vi "Get Installed Set Extended.vi"(8 "error in (no error)":errorcluster, 9 "Item Types (all visible)":T1 items=["all visible", "all including hidden", "standard only", "startup only"], 10 "Cached (F)":bool, 11 "Session in":refnum<k21>) -> (0 "error out":errorcluster, 2 "Software Set":T2 {"Items"."Visibility Type" items=["standard", "hidden", "system", "unknown", "startup", "image"]; "Add-ons"."Visibility Type" items=["standard", "hidden", "system", "unknown", "startup", "image"]}, 3 "Session out":refnum<k21>)   [LabVIEW 2012, in "nisyscfg.lvlib"]
uses:
  <vilib>/nisyscfg/nisyscfg.lvlib
  <vilib>/nisyscfg/Software Set Extended.ctl
  <vilib>/nisyscfg/Software Extended.ctl
  <vilib>/nisyscfg/Component Type.ctl
  <vilib>/nisyscfg/Component Types.ctl
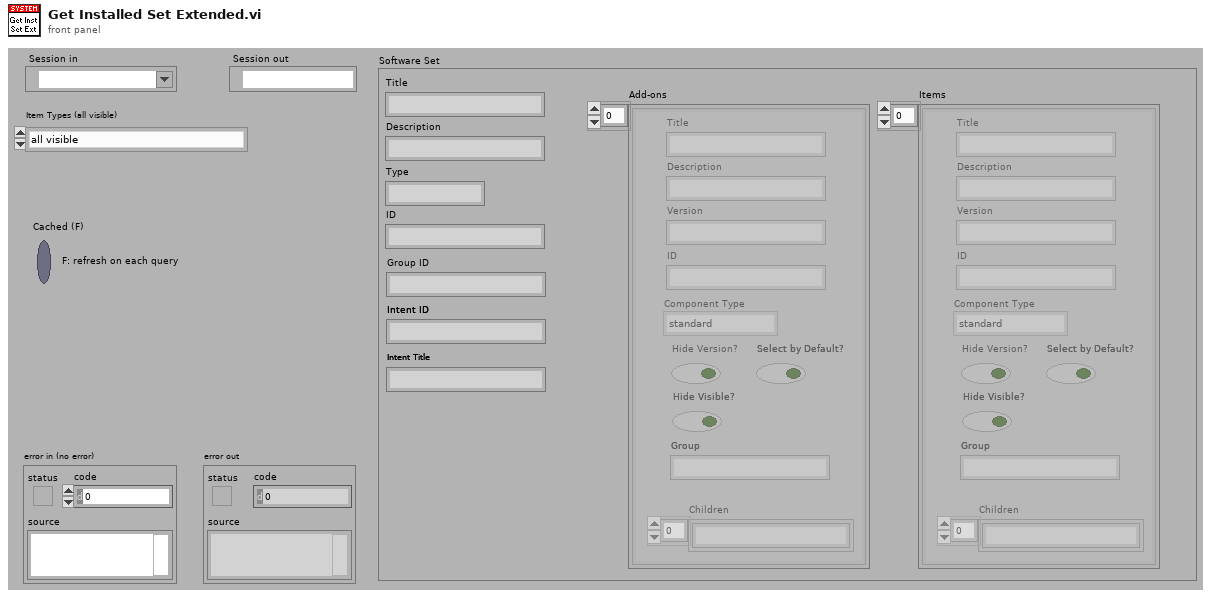
[diagram p1: front panel]
types:
  T1 = typedef "nisyscfg.lvlib/Component Types.ctl" = u32
  T2 = typedef "nisyscfg.lvlib/Software Set Extended.ctl" = cluster{"Description":string, "ID":string, "Type":string, "Title":string, "Add-ons":T3[], "Items":T3[], "Group ID":string, "Intent ID":string, "Intent Title":string}
  T3 = typedef "nisyscfg.lvlib/Software Extended.ctl" = cluster{"Description":string, "ID":string, "Version":string, "Title":string, "Visibility Type":T4, "Hide Version?":bool, "Children":string[], "Select by Default?":bool, "Hide Visible?":bool, "Group":string}
  T4 = typedef "nisyscfg.lvlib/Component Type.ctl" = u32
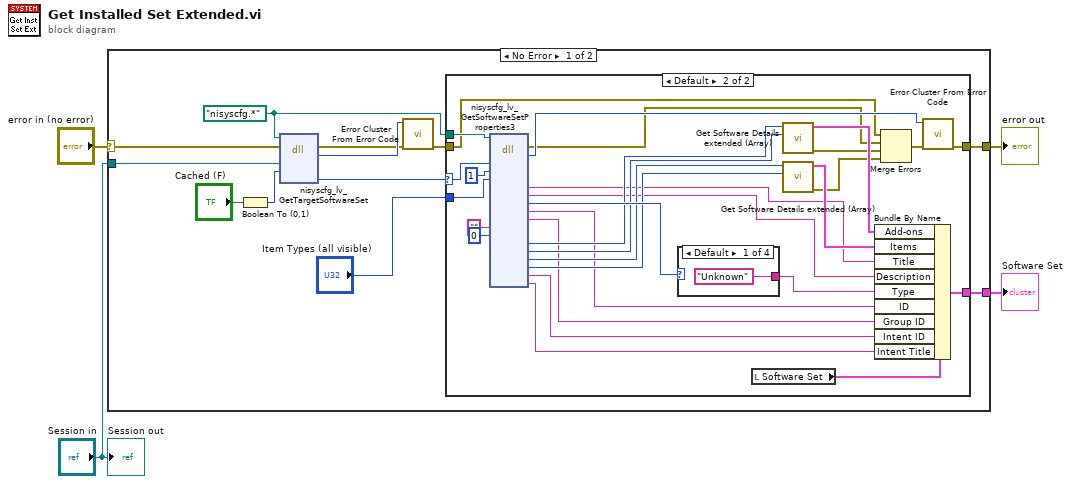
[diagram p0: block diagram]
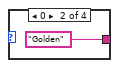
[diagram p3: hidden frame]
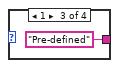
[diagram p4: hidden frame]
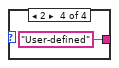
[diagram p5: hidden frame]
diagram:
  n1 = case shown="No Error" "error in (no error)" {
    selector: "error in (no error)" -> [w14 w51]
    tunnel: [w16 w51] -> w4
    tunnel: [w15 _] -> w1
    tunnel: "Session in" -> [w13 _]
    frame No Error {
      w12 = path "nisyscfg.*" ("path in")
      n2 = Boolean To (0,1)(Boolean="Cached (F)") -> (0, 1=w10:i16)
      n3 = dll-call lib="nisyscfg.*" fn="nisyscfg_lv_GetTargetSoftwareSet" label="GetTargetSoftwareSet"(path in=w12, error in=w14, "session"=w13, "cached"=w10) -> (error out=w7:errorcluster, "result"=w8:i32, "softwareSet"=w9:u64)  [unwired: 4 in, 1 out]
      n4 = call <vilib>:"Error Cluster From Error Code.vi"("error in (no error)"=w7, "error code (0)"=w8) -> ("error out"=w6:errorcluster)  [unwired: 7 in]
      n5 = case shown="Default" w9 {
        selector: w9 -> [_ w38]
        tunnel: w6 -> [w17 w26]
        tunnel: [w17 w27] -> w16
        tunnel: [_ w43] -> w15
        tunnel: w12 -> [_ w42]
        tunnel: "Item Types (all visible)" -> [_ w21]
        frame 0 {
        }
        frame Default {
          n6 = dll-call lib="nisyscfg.*" fn="nisyscfg_lv_GetSoftwareSetProperties3" label="GetSoftwareSetProperties3"(path in=w42, "set"=w38, "includeAddOnDeps"=u32 1, "includeTypes"=w21, "version"="", "visibleType"=0) -> (error out=w25:errorcluster, "result"=w44:i32, "title"=w30:string, "description"=w29:string, "type"=w45:u32, "ID"=w33:string, "groupID"=w32:string, "addons"=w41:u64, "numAddons"=w37:i32, "items"=w40:u64, "numItems"=w36:i32, "intentID"=w23:string, "intentTitle"=w22:string)  [unwired: 18 in, 1 out]
          n7 = case shown="Default" w45 {
            tunnel: ["Unknown" "Golden" "Pre-defined" "User-defined"] -> w31
            frame Default {
            }
            frame 0 {
            }
            frame 1 {
            }
            frame 2 {
            }
          }
          n8 = local read "Software Set"() -> (w39:T2)
          n9 = call <vilib>:"Get Software Details extended (Array).vi"("Number of Elements"=w37, "Enumerator in"=w41) -> ("error out"=w24:errorcluster, "Software Components"=w35:T3[])  [unwired: 8 in]
          n10 = call <vilib>:"Get Software Details extended (Array).vi"("Number of Elements"=w36, "Enumerator in"=w40) -> ("error out"=w18:errorcluster, "Software Components"=w34:T3[])  [unwired: 8 in]
          n11 = Bundle By Name(cluster=w39, "Add-ons"=w35, "Items"=w34, "Title"=w30, "Description"=w29, "Type"=w31, "ID"=w33, "Group ID"=w32, "Intent ID"=w23, "Intent Title"=w22) -> (w43:T2)
          n12 = Merge Errors(w26, w25, w24, w18) -> (w28:errorcluster)
          n13 = call <vilib>:"Error Cluster From Error Code.vi"("error in (no error)"=w28, "error code (0)"=w44) -> ("error out"=w27:errorcluster)  [unwired: 7 in]
        }
      }
    }
    frame Error {
    }
  }
  "error out" <- w4
  "Software Set" <- w1
  "Session out" <- "Session in"
